vi "SpecA_MXA_MatchIDNStr.vi"(8 "error in (no error)":errorcluster, 10 "IDNStr":string) -> (0 "error out":errorcluster, 2 "IDN match":bool, 3 "ClassLibraryFile":path)   [LabVIEW 2014]
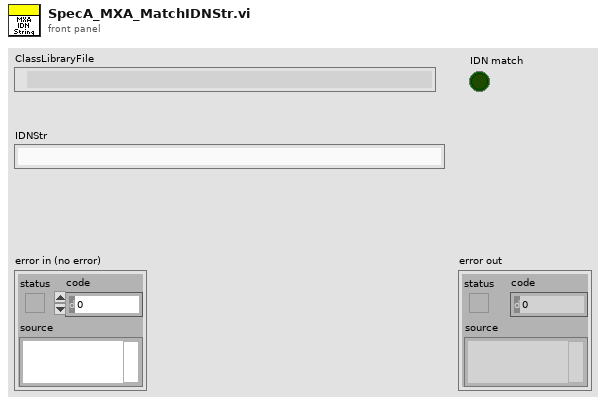
[diagram p1: front panel]
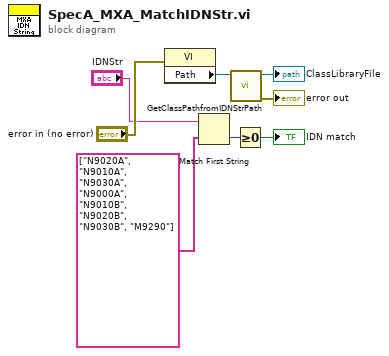
[diagram p0: block diagram]
diagram:
  n1 = property class="VI"(error in="error in (no error)") -> ("Path"=w6:path)  [unwired: 1 in, 2 out]
  n2 = Match First String(2:string[] ["N9020A", "N9010A", "N9030A", "N9000A", "N9010B", "N9020B", "N9030B", "M9290"], 3:"IDNStr") -> (0:w4:i32)  [unwired: 1 out]
  n3 = call "GetClassPathfromIDNStrPath.vi"("Path in"=w6) -> ("error out"=→"error out":errorcluster, "Path out"=→"ClassLibraryFile":path)  [unwired: 9 in]
  n4 = Greater Or Equal To 0?(x=w4) -> (x >= 0?=→"IDN match":bool)
